vi "slowcontrol3.vi"(6 "stop":bool, 7 "VISA resource name":refnum<visa-resource-name>="COM5", 8 "Write to file":bool=TRUE, 10 "IP Address of NIST Server":string="128.210.146.230", 11 "Output Directory":path) -> (0 "data":string[](array[string]), 3 "unix time stamp":u64)   [LabVIEW 2012]
uses:
  <vilib>/Platform/TimedLoop/XDataNode/timing_clust.ctl
  <vilib>/Platform/TimedLoop/XDataNode/nitl_modes.ctl
  <vilib>/Platform/TimedLoop/XDataNode/wakeup.ctl
  <vilib>/Platform/TimedLoop/TimeConversion.llb/rt-rel-time-to-milliseconds.vi
  <vilib>/Instr/_visa.llb/VISA Configure Serial Port (Instr).vi
  <vilib>/Platform/TimedLoop/XDataNode/XDataNode.xnode
  <vilib>/Platform/TimedLoop/XDataNode/XDNodeRunTimeDep.lvlib
panel:
  out "XML String":string
  in  "Array to specify the range":dbl[][](array[numeric])=[[1657984570.0, 30.0, 105000.0, 1000.0, 1000.0, 1000.0, 700.0, 100.0, 5.0], [1342904000.0, 20.0, 95000.0, -1000.0, -1000.0, -1000.0, 650.0, 0.0, 1.0]] format="%^#_10g"
  out "data with color code":cluster{"Color Box":u32, "String":string}[](array[cluster])
  out "mean value":dbl[](array[numeric])
  in  "Period [s]":dbl=10.0
  out "number of read-out\nvariables":i32
  out "names string":string
  out "parameternames":string
  out "date/time string":string
  out "array of datanames 2":string[](array[string])
  in  "XOFF Character":u8=19 format="%.0x"
  in  "XON Character":u8=17 format="%.0x"
  out "reinitialize arduino\nread boolean":bool
  out "Magnetic Field Z Coordinate":dbl(graph)
  out "Magnetic Field Y Coordinate":dbl(graph)
  out "Magnetic Field X Coordinate":dbl(graph)
  out "Total Magnetic Field":dbl(graph)
  out "Humidity":dbl(graph)
  out "Temperature":dbl(graph)
  out "Pressure":dbl(graph)
  in  "number of iterations to\nbuild mean value":i32=5
  out "array of datanames":string[](array[string])
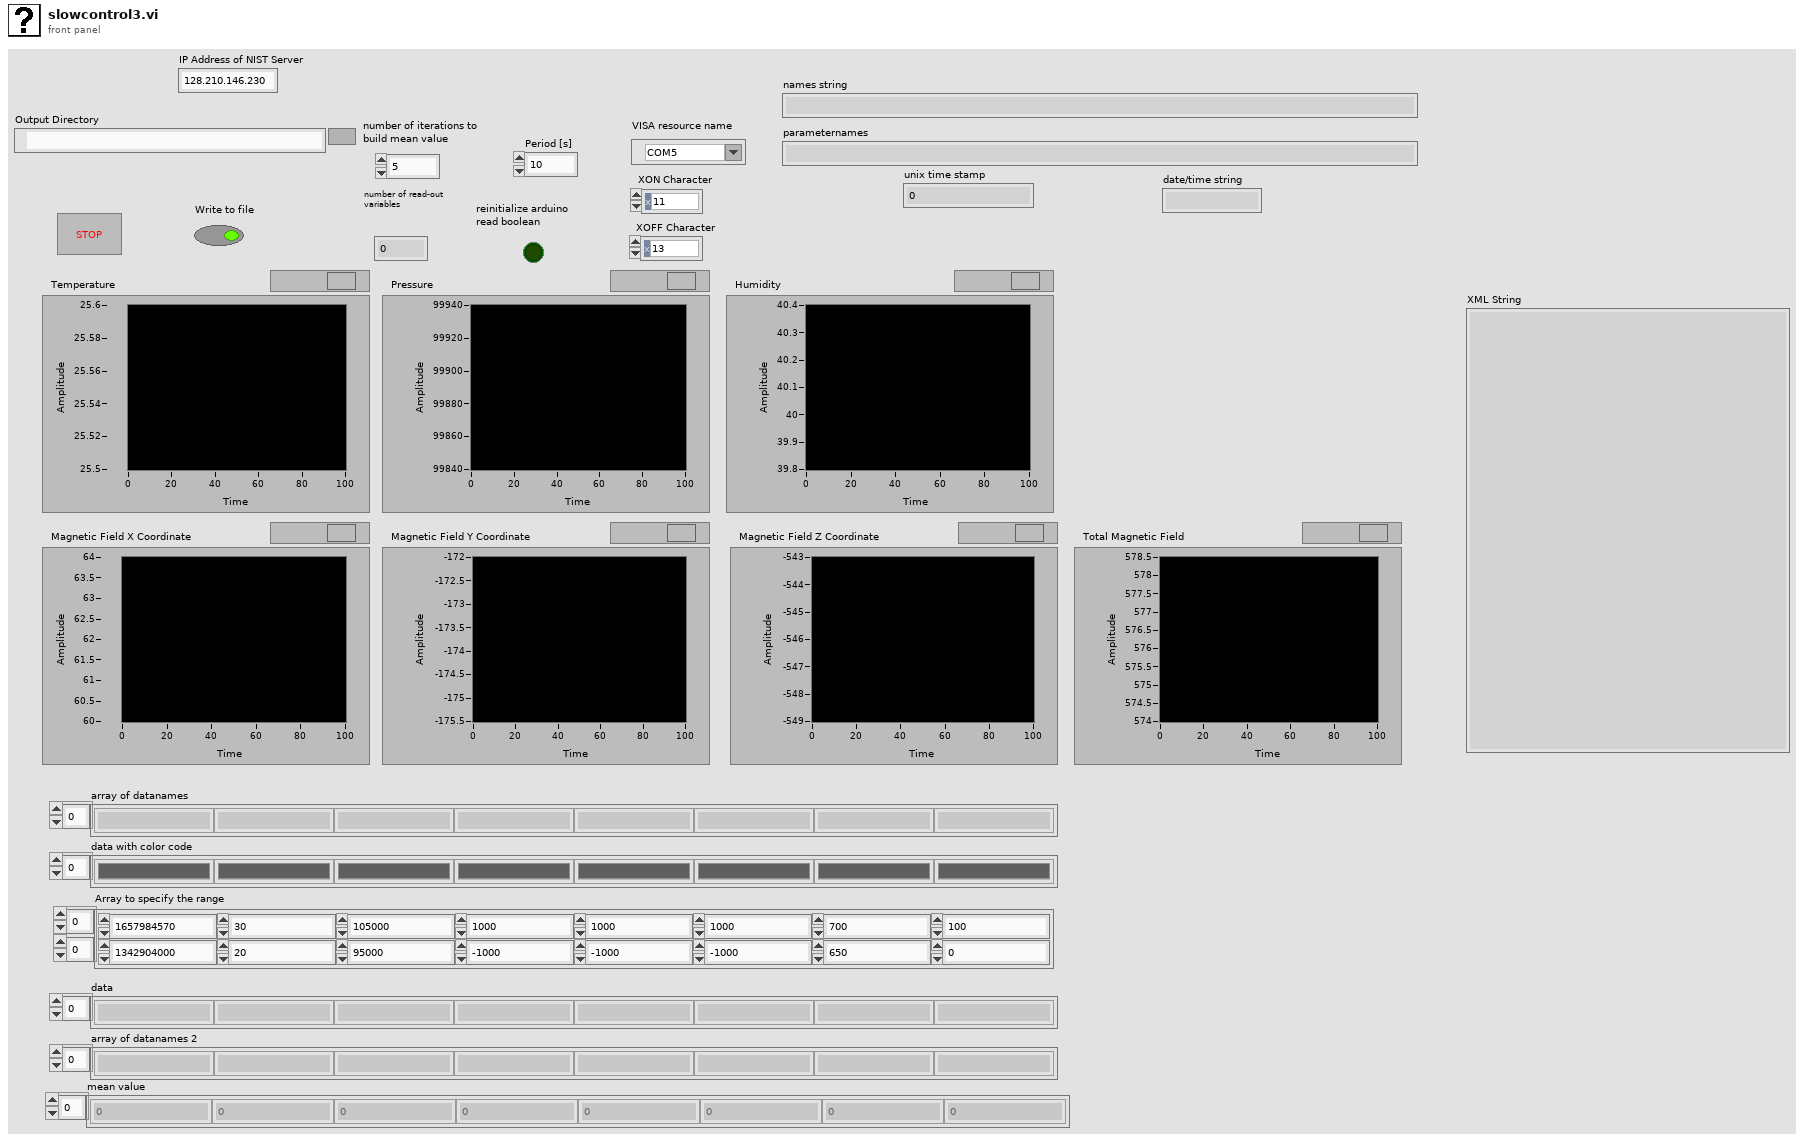
[diagram p1: front panel]
types:
  T1 = enum16{"open", "replace", "create", "open or create", "replace or create", "replace or create with confirmation"}
  T2 = typedef "XDNodeRunTimeDep.lvlib/timing_clust.ctl" = cluster{"Expected End [f-1]":u64, "Actual End [f-1]":u64, "Finished Late? [f-1]":bool, "Expected End [i-1]":u64, "Actual End [i-1]":u64, "Finished Late? [i-1]":bool, "Expected Start [i]":u64, "Actual Start [i]":u64, "Expected Start [f]":u64, "Actual Start [f]":u64, "Source Name":string, "Structure Name":string, "Period":i64, "Deadline":i64, "Offset":i64, "Start":i64, "Priority":i32, "Timeout":i32, "Mode":T3, "Wakeup Reason":T4, "Error":errorcluster, "Source Type":string, "Secondary Source Type":string, "Global End Time":u64, "Global Start Time":u64, "Frame Duration":u64, "Iteration Duration":u64, "Assigned CPU":i32, "I/O Scan Engine Mode":u32}
  T3 = typedef "XDNodeRunTimeDep.lvlib/nitl_modes.ctl" = enum32{"No Change", "Process missed periods, maintain original phase", "Discard missed periods, maintain original phase", "Process missed periods, ignore original phase", "Discard missed periods, ignore original phase"}
  T4 = typedef "XDNodeRunTimeDep.lvlib/wakeup.ctl" = enum32{"Normal", "Aborted", "Asynchronous wakeup", "Timing source error", "Timed loop error", "Timeout"}
  T5 = enum16{"big-endian, network order", "native, host order", "little-endian"}
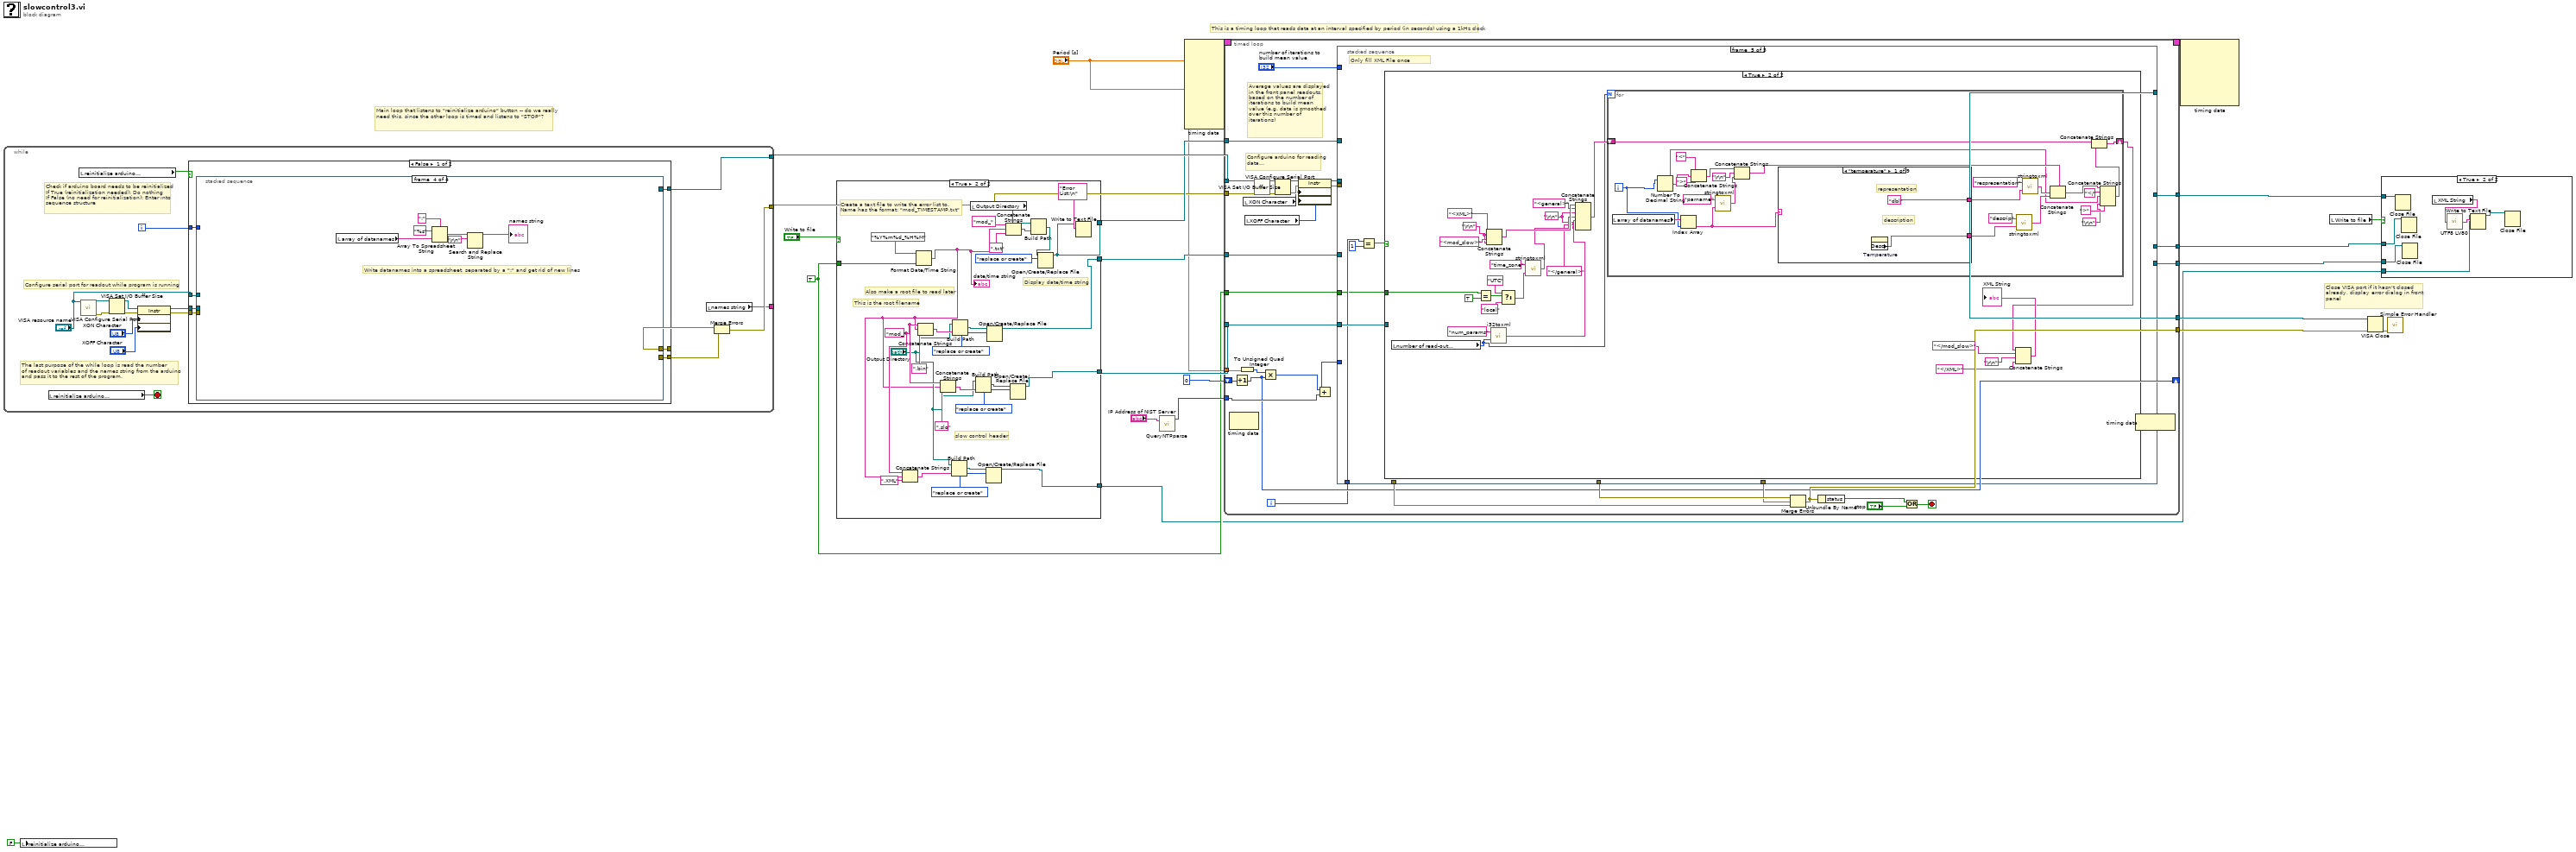
[diagram p0: block diagram]
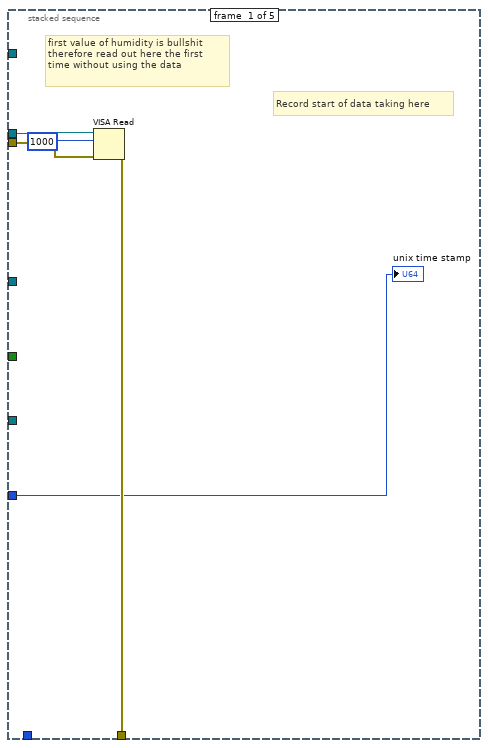
[diagram p4: hidden frame]
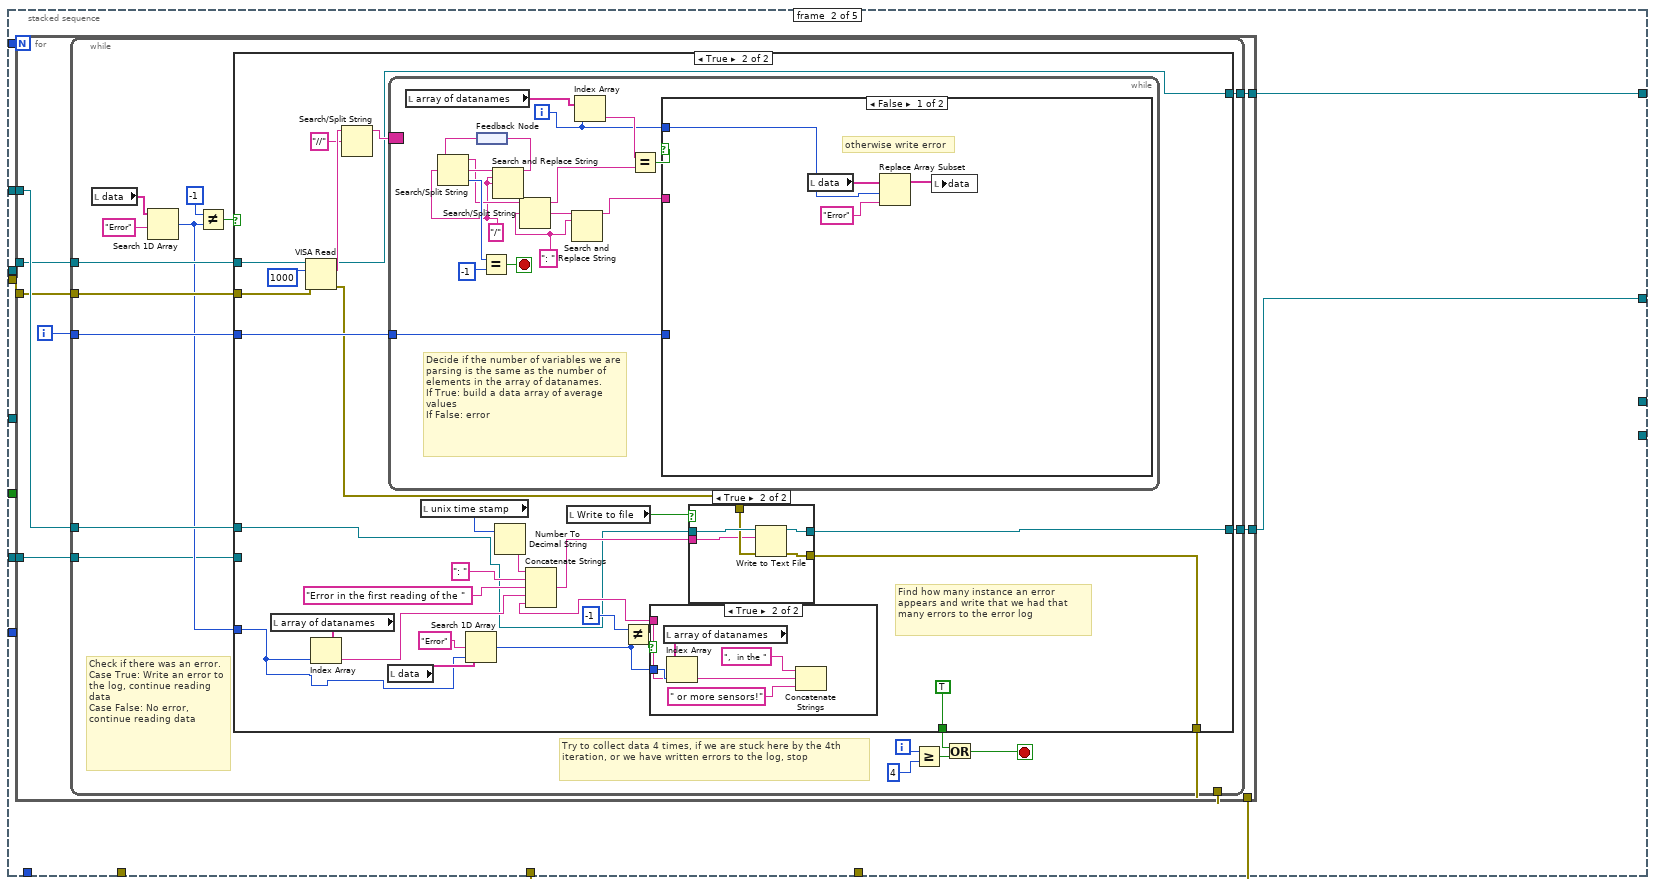
[diagram p5: hidden frame]
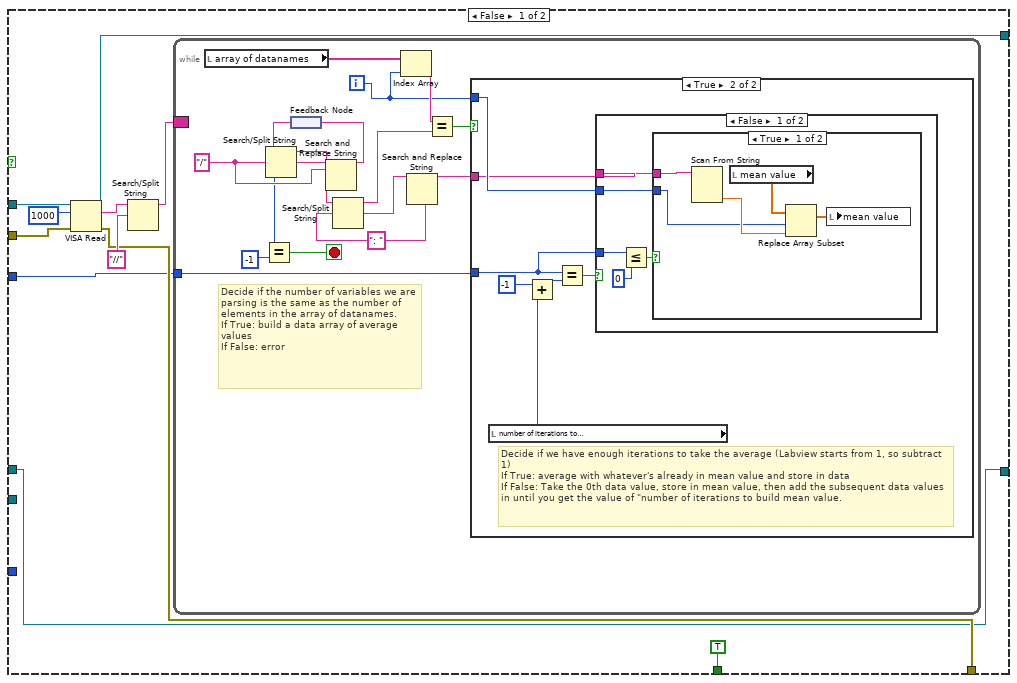
[diagram p6: hidden frame]
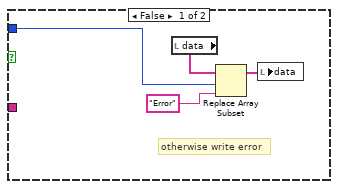
[diagram p7: hidden frame]
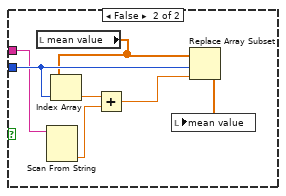
[diagram p8: hidden frame]
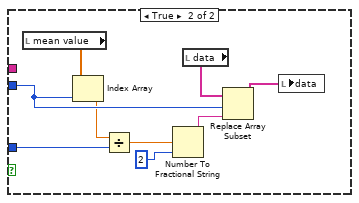
[diagram p9: hidden frame]
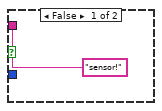
[diagram p11: hidden frame]
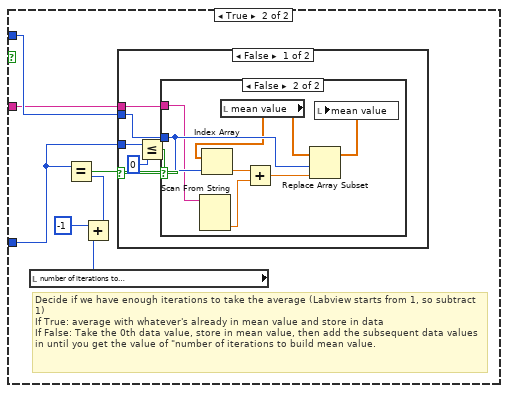
[diagram p12: hidden frame]
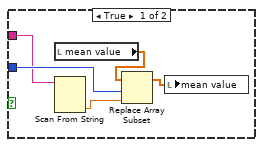
[diagram p13: hidden frame]
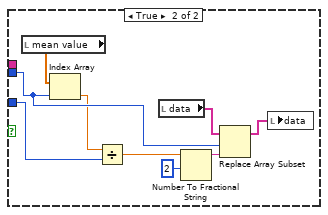
[diagram p14: hidden frame]
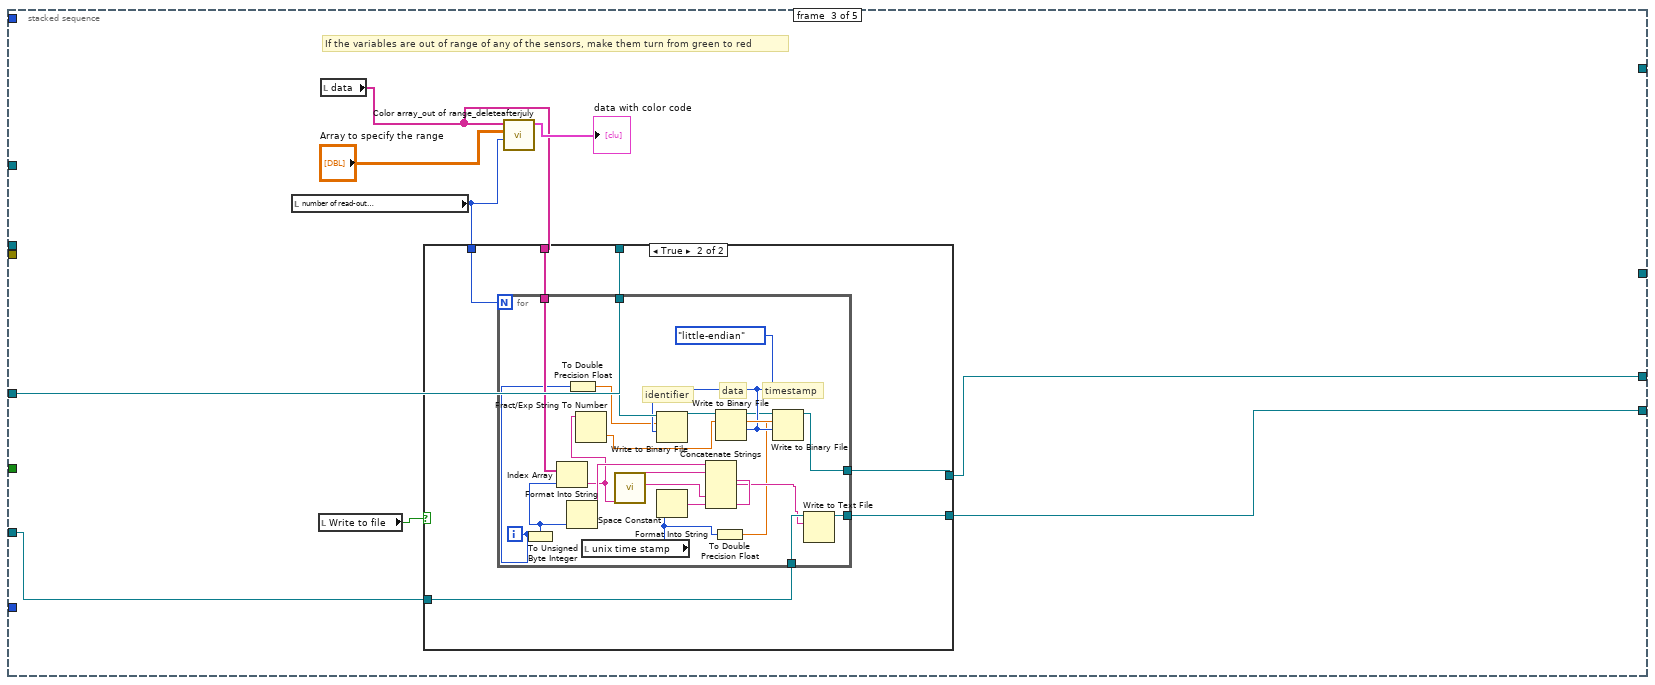
[diagram p15: hidden frame]
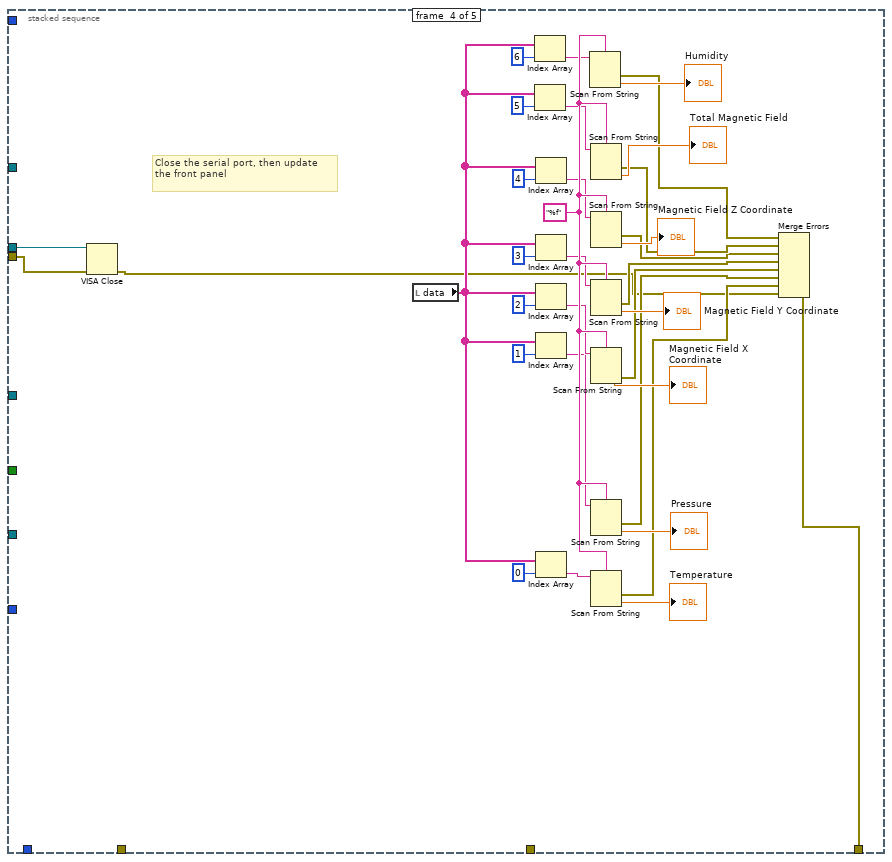
[diagram p17: hidden frame]
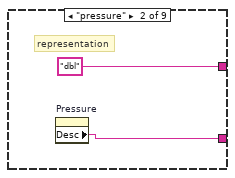
[diagram p19: hidden frame]
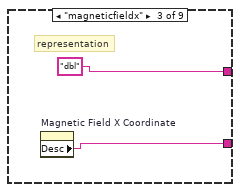
[diagram p20: hidden frame]
diagram:
  w2 = TRUE
  # "Main loop that listens to \"reinitialize arduino\" button -- do we really need this, since the other loop is timed and listens to \"STOP\"?"
  # "Close VISA port if it hasn't closed already, display error dialog in front panel"
  # "This is a timing loop that reads data at an interval specified by period (in seconds) using a 1kHz clock"
  n1 = while {
    tunnel: [w33] -> w22
    tunnel: [w32] -> w14
    tunnel: [w26] -> _
    i -> [w30]
    stop <- w28 stop-if-true
    # "The last purpose of the while loop is read the number \nof readout variables and the names string from the arduino\nand pass it to the rest of the program."
    # "Check if arduino board needs to be reinitialized\nIf True (reinitialization needed): Do nothing\nIf False (no need for reinitialization): Enter into \nsequence structure"
    # "Configure serial port for readout while program is running"
    n2 = local read "reinitialize arduino\nread boolean"() -> (w28:bool)
    n3 = local read "reinitialize arduino\nread boolean"() -> (w27:bool)
    n4 = call-poly "VISA Configure Serial Port"("VISA resource name"="VISA resource name") -> ("VISA resource name out"=w35:refnum<visa-resource-name>, "error out"=w34:errorcluster)  [unwired: 9 in, 4 out]
    n5 = VISA Set I/O Buffer Size(VISA resource name=w35, error in (no error)=w34) -> (VISA resource name out=w39:refnum<visa-resource-name>, error out=w38:errorcluster)  [unwired: 2 in]
    n6 = property class="Instr"(reference=w39, error in=w38, "Serial Settings:Flow Control XON Character"="XON Character", "Serial Settings:Flow Control XOFF Character"="XOFF Character") -> (reference out=w31:refnum<visa-resource-name>, error out=w25:errorcluster)
    n7 = case shown="False" w27 {
      tunnel: [w46 w118] -> w33
      tunnel: w31 -> [w45 w118]
      tunnel: w30 -> [w44 _]
      tunnel: "VISA resource name" -> [w43 _]
      tunnel: w25 -> [w42 _]
      tunnel: [w41 _] -> w24
      tunnel: [w40 _] -> w23
      frame False {
        n8 = stacked-sequence {
          tunnel: [_ w71 _ _] -> w46
          tunnel: w45 -> [_ w74 w91 _]
          tunnel: w44 -> [w51 _ _ _]
          tunnel: w43 -> [w48 _ _ _]
          tunnel: w42 -> [_ w72 w89 _]
          tunnel: [_ w61 _ _] -> w41
          tunnel: [_ _ w88 _] -> w40
          frame #0 {
            # "If, after 4 loop iterations, we are still here, the sensor reading must have failed??  \nSo, set the reinitialize arduino value to true and stop the program"
            # "number of runs to try to fill the array"
            n9 = Greater Or Equal?(x=w51, y=4) -> (x >= y?=w49:bool)
            n10 = case shown="True" w49 {
              tunnel: w48 -> [_ w52]
              frame False {
              }
              frame True {
                n11 = flat-sequence {
                  tunnel: w52 -> [w53]
                  frame #0 {
                    # "Report and error and close VISA"
                    n12 = VISA Close(VISA resource name=w53) -> ()  [unwired: 1 in, 1 out]
                    n13 = One Button Dialog(message="Read-out of the names of the sensors failed.\nProgram will be stopped") -> ()  [unwired: 1 in, 1 out]
                  }
                  frame #1 {
                    # "Stop the program"
                    n14 = Stop(stop? (T)=TRUE) -> ()
                  }
                }
              }
            }
            "reinitialize arduino\nread boolean" <- TRUE ("reinitialize arduino\nread boolean")
          }
          frame #1 {
            w58 = "" ("names string")
            # "The rest must be data, so there you go..."
            # "Count the number of names, \nis the number of read-out variables"
            # "Search for the \"//\" at the start of the file, \nindicates data names are here"
            # "Initialize the local variables: \nnames string\nparameternames"
            # "Read the first 1000 bytes, \noutput as a string"
            # "Initialize the array and set it to zero"
            n15 = local write "names string"(w58) -> ()
            n16 = VISA Read(VISA resource name=w74, byte count=u32 1000, error in (no error)=w72) -> (VISA resource name out=w71:refnum<visa-resource-name>, read buffer=w70:string, error out=w62:errorcluster)  [unwired: 1 out]
            n17 = Search/Split String(string=w70, search string/char (-)="//") -> (substring before match=w66:string)  [unwired: 1 in, 2 out]
            n18 = while {
              border: w66 -> [_]
              i -> [w75]
              stop <- w84 stop-if-true
              w80 = "/" ("search string/char (-)")
              # "Further separate names by \":\"'s?"
              # "When no more \"/\"s are found,\n end while loop"
              # "Names are separated by \"/\"s, so search\n for them but do not replace"
              # "Separate array names and put them into \nthe local variable \"array of datanames\""
              n19 = feedback #1() -> (w82:string)
              n20 = Search/Split String(string=w82, search string/char (-)=w80) -> (substring before match=w78:string, match + rest of string=w77:string, offset of match=w79:i32)  [unwired: 1 in]
              n21 = Search and Replace String(input string=w77, search string=w80) -> (result string=w81:string)  [unwired: 6 in, 3 out]
              n22 = feedback-in #1(w81) -> ()
              n23 = Equal?(x=w79, y=-1) -> (x = y?=w84:bool)
              n24 = Search/Split String(string=w78, search string/char (-)=": " ("format string")) -> (substring before match=w76:string)  [unwired: 1 in, 2 out]
              n25 = local read "array of datanames"() -> (w86:string[])
              n26 = Replace Array Subset(array=w86, new element=w76, index=w75) -> (w85:string[])
              n27 = local write "array of datanames"(w85) -> ()
            }
            n28 = Search and Replace String(replace all?=TRUE ("replace all? (F)"), input string=w66, search string="/", error in=w62) -> (number of replacements=w67:i32, error out=w61:errorcluster)  [unwired: 4 in, 2 out]
            n29 = Add(x=1, y=w67) -> (x+y=w57:i32)
            "number of read-out\nvariables" <- w57
            n30 = Initialize Array("", w57) -> (→"data" →"array of datanames" →"array of datanames 2":string[])
            n31 = Initialize Array(0.0 ("element"), w57) -> (→"mean value":dbl[])
            "parameternames" <- w58
          }
          frame #2 {
            # "Fill array of datanames 2 to check???\nIf they don't match, reinitialize."
            n32 = VISA Read(VISA resource name=w91, byte count=u32 1000, error in (no error)=w89) -> (read buffer=w94:string, error out=w88:errorcluster)  [unwired: 2 out]
            n33 = Search/Split String(string=w94, search string/char (-)="//") -> (substring before match=w90:string)  [unwired: 1 in, 2 out]
            n34 = while {
              border: w90 -> [_]
              i -> [w95]
              stop <- w106 stop-if-true
              w101 = "/" ("search string/char (-)")
              # "second output to manually\ncontrol the array"
              # "check if the name already exists"
              # "control the names in the array"
              n35 = local read "array of datanames 2"() -> (w108:string[])
              n36 = feedback #2() -> (w104:string)
              n37 = Search/Split String(string=w104, search string/char (-)=w101) -> (substring before match=w109:string, match + rest of string=w103:string, offset of match=w100:i32)  [unwired: 1 in]
              n38 = Search and Replace String(input string=w103, search string=w101) -> (result string=w102:string)  [unwired: 6 in, 3 out]
              n39 = feedback-in #2(w102) -> ()
              n40 = Search/Split String(string=w109, search string/char (-)=": " ("format string")) -> (substring before match=w97:string)  [unwired: 1 in, 2 out]
              n41 = Equal?(x=w100, y=-1) -> (x = y?=w106:bool)
              n42 = local read "array of datanames"() -> (w98:string[])
              n43 = Replace Array Subset(array=w108, new element=w97, index=w95) -> (w107:string[])
              n44 = local write "array of datanames 2"(w107) -> ()
              n45 = Index Array(array=w98, index=w95) -> (element=w99:string)
              n46 = Equal?(x=w99, y=w97) -> (x = y?=w96:bool)
              n47 = case shown="False" w96 {
                frame False {
                  n48 = local write "reinitialize arduino\nread boolean"(FALSE ("reinitialize arduino read boolean")) -> ()
                }
                frame True {
                }
              }
            }
          }
          frame #3 {
            # "Write datanames into a spreadsheet, separated by a \":\" and get rid of new lines"
            n49 = local read "array of datanames"() -> (w117:string[])
            n50 = Array To Spreadsheet String(delimiter (Tab)=":", array=w117, 3:"%s" ("format string")) -> (spreadsheet string=w113:string)
            n51 = Search and Replace String(input string=w113, search string="\r\n") -> (result string=→"names string":string)  [unwired: 6 in, 3 out]
          }
        }
      }
      frame True {
      }
    }
    n52 = local read "names string"() -> (w26:string)
    n53 = Merge Errors(w24, w23) -> (w32:errorcluster)
  }
  n54 = local write "reinitialize arduino\nread boolean"(FALSE ("reinitialize arduino\nread boolean")) -> ()
  n55 = case shown="True" "Write to file" {
    tunnel: [_ w141] -> w18
    tunnel: [_ w130] -> w13
    tunnel: [_ w129] -> w4
    tunnel: [_ w122] -> w1
    tunnel: w2 -> [_ w119]
    frame False {
    }
    frame True {
      w126 = "mod_"
      # "slow control header"
      # "This is the root filename"
      # "Display date/time string"
      # "Also make a root file to read later"
      # "Create a text file to write the error list to.  \nName has the format: \"mod_TIMESTAMP.txt\""
      n56 = Format Date/Time String(time format string (%c)="%Y%m%d_%H%M", UTC format=w119) -> (date/time string=w120:string)  [unwired: 1 in]
      "date/time string" <- w120
      n57 = Concatenate Strings(w126, w120, ".XML" ("string")) -> (w124:string)
      n58 = Concatenate Strings(w126, w120, ".bin") -> (w139:string)
      n59 = Concatenate Strings(w126, w120, ".slo") -> (w131:string)
      n60 = Build Path(base path="Output Directory", name or relative path=w124) -> (appended path=w127:path)
      n61 = Build Path(base path="Output Directory", name or relative path=w139) -> (appended path=w138:path)
      n62 = local read "Output Directory"() -> (w137:path)
      n63 = Build Path(base path="Output Directory", name or relative path=w131) -> (appended path=w132:path)
      n64 = Open/Create/Replace File(file path (use dialog)=w127, operation (0:open)=T1."replace or create") -> (refnum out=w122:refnum<file>)  [unwired: 4 in, 2 out]
      n65 = Open/Create/Replace File(file path (use dialog)=w138, operation (0:open)=T1."replace or create") -> (refnum out=w130:refnum<file>)  [unwired: 4 in, 2 out]
      n66 = Concatenate Strings("mod_", w120, ".txt") -> (w136:string)
      n67 = Open/Create/Replace File(file path (use dialog)=w132, operation (0:open)=T1."replace or create") -> (refnum out=w129:refnum<file>)  [unwired: 4 in, 2 out]
      n68 = Build Path(base path=w137, name or relative path=w136) -> (appended path=w135:path)
      n69 = Open/Create/Replace File(file path (use dialog)=w135, operation (0:open)=T1."replace or create") -> (refnum out=w141:refnum<file>)  [unwired: 4 in, 2 out]
      n70 = Write to Text File(file (use dialog)=w141, text="Error List:\n") -> ()  [unwired: 2 in, 3 out]
    }
  }
  n71 = call "QueryNTPparse.vi"("Hostname"="IP Address of NIST Server") -> ("NTP Time"=w5:u64)  [unwired: 1 in, 2 out]
  n72 = node-c288("Period [s]") -> (w21:T2)  [unwired: 9 in]
  n73 = timed-loop {
    tunnel: w22 -> [w173]
    tunnel: w14 -> [w171]
    tunnel: [w174] -> w15
    timing: w21 -> [_]
    timing-out: [_] -> w20
    tunnel: w18 -> [w175]
    tunnel: [w163] -> w16
    tunnel: w13 -> [w160]
    tunnel: [w149] -> w12
    tunnel: [w159] -> w11
    tunnel: w5 -> [w157]
    shift-right: [w152] -> _
    shift-left: u64 0 -> [w158]
    tunnel: "Period [s]" -> [w155]
    tunnel: w4 -> [w151]
    tunnel: [w150] -> w3
    tunnel: w2 -> [w147]
    i -> [w148]
    stop <- w178 stop-if-true
    # "Configure arduino for reading data..."
    # "Average values are displayed in the front panel readouts, based on the number of iterations to build mean value (e.g. data is smoothed over this number of iterations)"
    n74 = node-c288() -> ()  [unwired: 1 in, 1 out]
    n75 = Increment(x=w158) -> (x+1=w152:u64)
    n76 = To Unsigned Quad Integer(1:w155) -> (0:w154:u64)
    n77 = local read "XON Character"() -> (w164:u8)
    n78 = local read "XOFF Character"() -> (w165:u8)
    n79 = call-poly "VISA Configure Serial Port"("VISA resource name"=w173, "error in (no error)"=w171) -> ("VISA resource name out"=w172:refnum<visa-resource-name>, "error out"=w170:errorcluster)  [unwired: 8 in, 4 out]
    n80 = Multiply(x=w154, y=w152) -> (x*y=w153:u64)
    n81 = VISA Set I/O Buffer Size(VISA resource name=w172, error in (no error)=w170) -> (VISA resource name out=w166:refnum<visa-resource-name>, error out=w169:errorcluster)  [unwired: 2 in]
    n82 = property class="Instr"(reference=w166, error in=w169, "Serial Settings:Flow Control XON Character"=w164, "Serial Settings:Flow Control XOFF Character"=w165) -> (reference out=w167:refnum<visa-resource-name>, error out=w168:errorcluster)
    n83 = Add(x=w153, y=w157) -> (x+y=w156:u64)
    n84 = stacked-sequence {
      tunnel: [_ _ _ w420 _] -> w176
      tunnel: [_ w192 _ _ _] -> w177
      tunnel: w175 -> [_ w193 _ _ _]
      tunnel: w168 -> [w186 w195 _ w418 _]
      tunnel: w167 -> [w187 w194 _ w419 _]
      tunnel: [_ w191 _ _ _] -> w163
      tunnel: "number of iterations to\nbuild mean value" -> [_ w190 _ _ _]
      tunnel: [w184 _ _ _ _] -> w161
      tunnel: w160 -> [_ _ w388 _ _]
      tunnel: [_ _ w389 _ _] -> w159
      tunnel: w156 -> [w183 _ _ _ _]
      tunnel: w151 -> [_ w189 w384 _ w455]
      tunnel: [_ _ w383 _ _] -> w150
      tunnel: [_ w188 _ _ _] -> w149
      tunnel: w148 -> [_ _ _ _ w453]
      tunnel: w147 -> [_ _ _ _ w451]
      frame #0 {
        # "first value of humidity is bullshit therefore read out here the first time without using the data"
        # "Record start of data taking here"
        n85 = VISA Read(VISA resource name=w187, byte count=u32 1000, error in (no error)=w186) -> (error out=w184:errorcluster)  [unwired: 3 out]
        "unix time stamp" <- w183
      }
      frame #1 {
        n86 = for {
          N: w190 -> [_]
          tunnel: w195 -> [w200]
          tunnel: w194 -> [w201]
          tunnel: w193 -> [w203]
          tunnel: [w202] -> w192
          tunnel: [w199] -> w191
          tunnel: [w197] -> w188
          tunnel: w189 -> [w196]
          i -> [w198]
          n87 = while {
            tunnel: w203 -> [w215]
            tunnel: [w214] -> w202
            tunnel: w201 -> [w213]
            tunnel: w200 -> [w211]
            tunnel: [w212] -> w199
            tunnel: w198 -> [w210]
            tunnel: [w207] -> w197
            tunnel: w196 -> [w204]
            i -> [w220]
            stop <- w216 stop-if-true
            # "Try to collect data 4 times, if we are stuck here by the 4th iteration, or we have written errors to the log, stop"
            # "Check if there was an error.  \nCase True: Write an error to the log, continue reading data\nCase False: No error, continue reading data"
            n88 = local read "data"() -> (w206:string[])
            n89 = Search 1D Array(1D array=w206, element="Error") -> (index of element=w208:i32)  [unwired: 1 in]
            n90 = Not Equal?(x=-1 ("y"), y=w208) -> (x != y?=w205:bool)
            n91 = case shown="True" w205 {
              tunnel: w208 -> [_ w289]
              tunnel: [TRUE TRUE] -> w217
              tunnel: w215 -> [w222 w297]
              tunnel: [w224 w296] -> w214
              tunnel: w213 -> [w227 w295]
              tunnel: [w226 w294] -> w212
              tunnel: w211 -> [w225 w293]
              tunnel: w210 -> [w223 w292]
              tunnel: [w222 w290] -> w207
              tunnel: w204 -> [_ _]
              frame False {
                n92 = VISA Read(VISA resource name=w227, byte count=u32 1000, error in (no error)=w225) -> (VISA resource name out=w226:refnum<visa-resource-name>, read buffer=w228:string, error out=w224:errorcluster)  [unwired: 1 out]
                n93 = Search/Split String(string=w228, search string/char (-)="//") -> (substring before match=w231:string)  [unwired: 1 in, 2 out]
                n94 = while {
                  border: w231 -> [_]
                  tunnel: w223 -> [w234]
                  i -> [w233]
                  stop <- w249 stop-if-true
                  w237 = ": " ("format string")
                  w244 = "/" ("search string/char (-)")
                  # "Decide if the number of variables we are parsing is the same as the number of elements in the array of datanames.  \nIf True: build a data array of average values\nIf False: error"
                  n95 = local read "array of datanames"() -> (w240:string[])
                  n96 = feedback #3() -> (w247:string)
                  n97 = Search/Split String(string=w247, search string/char (-)=w244) -> (substring before match=w238:string, match + rest of string=w246:string, offset of match=w243:i32)  [unwired: 1 in]
                  n98 = Equal?(x=w243, y=-1) -> (x = y?=w249:bool)
                  n99 = Search and Replace String(input string=w246, search string=w244) -> (result string=w245:string)  [unwired: 6 in, 3 out]
                  n100 = feedback-in #3(w245) -> ()
                  n101 = Search/Split String(string=w238, search string/char (-)=w237) -> (substring before match=w242:string, match + rest of string=w239:string)  [unwired: 1 in, 1 out]
                  n102 = Index Array(array=w240, index=w233) -> (element=w241:string)
                  n103 = Search and Replace String(input string=w239, search string=w237) -> (result string=w235:string)  [unwired: 6 in, 3 out]
                  n104 = Equal?(x=w241, y=w242) -> (x = y?=w236:bool)
                  n105 = case shown="True" w236 {
                    tunnel: w235 -> [_ w259]
                    tunnel: w233 -> [w253 w260]
                    tunnel: w234 -> [_ w257]
                    frame False {
                      # "otherwise write error"
                      n106 = local read "data"() -> (w252:string[])
                      n107 = Replace Array Subset(array=w252, new element="Error" ("new element/subarray"), index=w253) -> (w251:string[])
                      n108 = local write "data"(w251) -> ()
                    }
                    frame True {
                      # "Decide if we have enough iterations to take the average (Labview starts from 1, so subtract 1)\nIf True: average with whatever's already in mean value and store in data\nIf False: Take the 0th data value, store in mean value, then add the subsequent data values in until you get the value of \"number of iterations to build mean value."
                      n109 = local read "number of iterations to\nbuild mean value"() -> (w256:i32)
                      n110 = Add(x=-1, y=w256) -> (x+y=w255:i32)
                      n111 = Equal?(x=w257, y=w255) -> (x = y?=w258:bool)
                      n112 = case shown="False" w258 {
                        tunnel: w257 -> [w265 w282]
                        tunnel: w260 -> [w262 w285]
                        tunnel: w259 -> [w261 _]
                        frame False {
                          n113 = Less Or Equal?(x=w265, y=0) -> (x <= y?=w264:bool)
                          n114 = case shown="True" w264 {
                            tunnel: w262 -> [w266 w276]
                            tunnel: w261 -> [w270 w275]
                            frame True {
                              n115 = Scan From String(input string=w270) -> (output 1=w269:dbl)  [unwired: 4 in, 3 out]
                              n116 = local read "mean value"() -> (w268:dbl[])
                              n117 = Replace Array Subset(array=w268, new element=w269, index=w266) -> (w267:dbl[])
                              n118 = local write "mean value"(w267) -> ()
                            }
                            frame False {
                              n119 = local read "mean value"() -> (w271:dbl[])
                              n120 = Scan From String(input string=w275) -> (output 1=w274:dbl)  [unwired: 4 in, 3 out]
                              n121 = Index Array(array=w271, index=w276) -> (element=w272:dbl)
                              n122 = Add(x=w272, y=w274) -> (x+y=w273:dbl)
                              n123 = Replace Array Subset(array=w271, new element=w273, index=w276) -> (w277:dbl[])
                              n124 = local write "mean value"(w277) -> ()
                            }
                          }
                        }
                        frame True {
                          n125 = local read "mean value"() -> (w279:dbl[])
                          n126 = Index Array(array=w279, index=w285) -> (element=w278:dbl)
                          n127 = Divide(x=w278, y=w282) -> (x/y=w283:dbl)
                          n128 = Number To Fractional String(number=w283, precision (6)=i16 2) -> (F-format string=w286:string)  [unwired: 2 in]
                          n129 = local read "data"() -> (w284:string[])
                          n130 = Replace Array Subset(array=w284, new element=w286, index=w285) -> (w281:string[])
                          n131 = local write "data"(w281) -> ()
                        }
                      }
                    }
                  }
                }
              }
              frame True {
                # "Find how many instance an error appears and write that we had that many errors to the error log"
                n132 = local read "array of datanames"() -> (w307:string[])
                n133 = VISA Read(VISA resource name=w295, byte count=u32 1000, error in (no error)=w293) -> (VISA resource name out=w294:refnum<visa-resource-name>, read buffer=w314:string, error out=w291:errorcluster)  [unwired: 1 out]
                n134 = Index Array(array=w307, index=w289) -> (element=w306:string)
                n135 = Search/Split String(string=w314, search string/char (-)="//") -> (substring before match=w311:string)  [unwired: 1 in, 2 out]
                n136 = local read "data"() -> (w305:string[])
                n137 = while {
                  border: w311 -> [_]
                  tunnel: w292 -> [w331]
                  i -> [w329]
                  stop <- w345 stop-if-true
                  w332 = ": " ("format string")
                  w330 = "/" ("search string/char (-)")
                  # "Decide if the number of variables we are parsing is the same as the number of elements in the array of datanames.  \nIf True: build a data array of average values\nIf False: error"
                  n138 = local read "array of datanames"() -> (w335:string[])
                  n139 = feedback #4() -> (w343:string)
                  n140 = Search/Split String(string=w343, search string/char (-)=w330) -> (substring before match=w333:string, match + rest of string=w342:string, offset of match=w340:i32)  [unwired: 1 in]
                  n141 = Equal?(x=w340, y=-1) -> (x = y?=w345:bool)
                  n142 = Search and Replace String(input string=w342, search string=w330, replace string=w330) -> (result string=w341:string)  [unwired: 5 in, 3 out]
                  n143 = feedback-in #4(w341) -> ()
                  n144 = Search/Split String(string=w333, search string/char (-)=w332) -> (substring before match=w338:string, match + rest of string=w334:string)  [unwired: 1 in, 1 out]
                  n145 = Search and Replace String(input string=w334, search string=w332) -> (result string=w339:string)  [unwired: 6 in, 3 out]
                  n146 = Index Array(array=w335, index=w329) -> (element=w337:string)
                  n147 = Equal?(x=w337, y=w338) -> (x = y?=w336:bool)
                  n148 = case shown="False" w336 {
                    tunnel: w339 -> [_ w355]
                    tunnel: w329 -> [w349 w356]
                    tunnel: w331 -> [_ w353]
                    frame False {
                      # "otherwise write error"
                      n149 = local read "data"() -> (w348:string[])
                      n150 = Replace Array Subset(array=w348, new element="Error" ("new element/subarray"), index=w349) -> (w347:string[])
                      n151 = local write "data"(w347) -> ()
                    }
                    frame True {
                      # "Decide if we have enough iterations to take the average (Labview starts from 1, so subtract 1)\nIf True: average with whatever's already in mean value and store in data\nIf False: Take the 0th data value, store in mean value, then add the subsequent data values in until you get the value of \"number of iterations to build mean value."
                      n152 = local read "number of iterations to\nbuild mean value"() -> (w352:i32)
                      n153 = Add(x=-1, y=w352) -> (x+y=w351:i32)
                      n154 = Equal?(x=w353, y=w351) -> (x = y?=w354:bool)
                      n155 = case shown="False" w354 {
                        tunnel: w353 -> [w361 w380]
                        tunnel: w356 -> [w358 w382]
                        tunnel: w355 -> [w357 _]
                        frame False {
                          n156 = Less Or Equal?(x=w361, y=0) -> (x <= y?=w360:bool)
                          n157 = case shown="False" w360 {
                            tunnel: w358 -> [w363 w372]
                            tunnel: w357 -> [w362 w371]
                            frame True {
                              n158 = local read "mean value"() -> (w365:dbl[])
                              n159 = Scan From String(input string=w362) -> (output 1=w366:dbl)  [unwired: 4 in, 3 out]
                              n160 = Replace Array Subset(array=w365, new element=w366, index=w363) -> (w364:dbl[])
                              n161 = local write "mean value"(w364) -> ()
                            }
                            frame False {
                              n162 = Scan From String(input string=w371) -> (output 1=w370:dbl)  [unwired: 4 in, 3 out]
                              n163 = local read "mean value"() -> (w367:dbl[])
                              n164 = Index Array(array=w367, index=w372) -> (element=w369:dbl)
                              n165 = Add(x=w369, y=w370) -> (x+y=w368:dbl)
                              n166 = Replace Array Subset(array=w367, new element=w368, index=w372) -> (w373:dbl[])
                              n167 = local write "mean value"(w373) -> ()
                            }
                          }
                        }
                        frame True {
                          n168 = local read "mean value"() -> (w374:dbl[])
                          n169 = Index Array(array=w374, index=w382) -> (element=w376:dbl)
                          n170 = Divide(x=w376, y=w380) -> (x/y=w375:dbl)
                          n171 = local read "data"() -> (w381:string[])
                          n172 = Number To Fractional String(number=w375, precision (6)=i16 2) -> (F-format string=w378:string)  [unwired: 2 in]
                          n173 = Replace Array Subset(array=w381, new element=w378, index=w382) -> (w379:string[])
                          n174 = local write "data"(w379) -> ()
                        }
                      }
                    }
                  }
                }
                n175 = local read "unix time stamp"() -> (w287:u64)
                n176 = Search 1D Array(1D array=w305, element="Error", start index (0)=w289) -> (index of element=w301:i32)
                n177 = Number To Decimal String(number=w287) -> (decimal integer string=w310:string)  [unwired: 1 in]
                n178 = local read "Write to file"() -> (w288:bool)
                n179 = Not Equal?(x=-1 ("y"), y=w301) -> (x != y?=w303:bool)
                n180 = case shown="True" w303 {
                  tunnel: w301 -> [_ w327]
                  tunnel: ["sensor!" w323] -> w300
                  frame False {
                  }
                  frame True {
                    n181 = local read "array of datanames"() -> (w328:string[])
                    n182 = Index Array(array=w328, index=w327) -> (element=w325:string)
                    n183 = Concatenate Strings(",  in the " ("string"), w325, " or more sensors!" ("string")) -> (w323:string)
                  }
                }
                n184 = Concatenate Strings(w310, ": ", "Error in the first reading of the ", w306, w300) -> (w299:string)
                n185 = case shown="True" w288 {
                  tunnel: w299 -> [_ w317]
                  tunnel: w297 -> [w316 w321]
                  tunnel: [w315 w320] -> w296
                  tunnel: w291 -> [w315 w319]
                  tunnel: [w316 w318] -> w290
                  frame False {
                  }
                  frame True {
                    n186 = Write to Text File(file (use dialog)=w321, text=w317, error in=w319) -> (refnum out=w318:refnum<file>, error out=w320:errorcluster)  [unwired: 1 in, 1 out]
                  }
                }
              }
            }
            n187 = Greater Or Equal?(x=w220, y=4) -> (x >= y?=w218:bool)
            n188 = Or(x=w217, y=w218) -> (x .or. y?=w216:bool)
          }
        }
      }
      frame #2 {
        # "If the variables are out of range of any of the sensors, make them turn from green to red"
        n189 = local read "number of read-out\nvariables"() -> (w386:i32)
        n190 = local read "Write to file"() -> (w385:bool)
        n191 = local read "data"() -> (w387:string[])
        n192 = case shown="True" w385 {
          tunnel: [_ w397] -> w389
          tunnel: w388 -> [_ w396]
          tunnel: w387 -> [_ w395]
          tunnel: w386 -> [_ w394]
          tunnel: [_ w393] -> w383
          tunnel: w384 -> [_ w392]
          frame False {
          }
          frame True {
            n193 = for {
              N: w394 -> [_]
              tunnel: [w400] -> w397
              tunnel: w396 -> [w409]
              tunnel: w395 -> [w416]
              tunnel: [w411] -> w393
              tunnel: w392 -> [w410]
              i -> [w402]
              w405 = T5."little-endian" ("byte order (0:big-endian, network order)")
              # "timestamp"
              # "data"
              # "identifier"
              n194 = To Unsigned Byte Integer(number=w402) -> (unsigned 8bit integer=w412:u8)
              n195 = Index Array(array=w416, index=w412) -> (element=w408:string)
              n196 = Format Into String(w412) -> (resulting string=w415:string)  [unwired: 3 in, 1 out]
              n197 = To Double Precision Float(number=w402) -> (double precision float=w401:dbl)
              n198 = Fract/Exp String To Number(string=w408) -> (number=w407:dbl)  [unwired: 3 in, 1 out]
              n199 = local read "unix time stamp"() -> (w404:u64)
              n200 = call <vilib>:"Space Constant.vi"() -> ("String"=w413:string)
              n201 = Write to Binary File(file (use dialog)=w409, data=w401, 9:w405) -> (refnum out=w398:refnum<file>)  [unwired: 3 in, 2 out]
              n202 = Format Into String(w404) -> (resulting string=w414:string)  [unwired: 3 in, 1 out]
              n203 = Concatenate Strings(w415, w413, w414, w413, w408, w413) -> (w406:string)
              n204 = To Double Precision Float(number=w404) -> (double precision float=w403:dbl)
              n205 = Write to Binary File(file (use dialog)=w398, data=w403, 9:w405) -> (refnum out=w399:refnum<file>)  [unwired: 3 in, 2 out]
              n206 = Write to Binary File(file (use dialog)=w399, data=w407, 9:w405) -> (refnum out=w400:refnum<file>)  [unwired: 3 in, 2 out]
              n207 = Write to Text File(file (use dialog)=w410, text=w406) -> (refnum out=w411:refnum<file>)  [unwired: 2 in, 2 out]
            }
          }
        }
        n208 = call "Color array_out of range_deleteafterjuly.vi"("Number of sensors"=w386, "Array to specify\nthe range"="Array to specify the range", "Input Array"=w387) -> ("output array with color code"=→"data with color code":cluster{"Color Box":u32, "String":string}[])  [unwired: 7 in, 1 out]
      }
      frame #3 {
        w434 = "%f" ("format string")
        # "Close the serial port, then update the front panel"
        n209 = VISA Close(VISA resource name=w419, error in (no error)=w418) -> (error out=w417:errorcluster)
        n210 = local read "data"() -> (w443:string[])
        n211 = Index Array(array=w443, index=6) -> (element=w428:string)
        n212 = Index Array(array=w443, index=5) -> (element=w429:string)
        n213 = Index Array(array=w443, index=4) -> (element=w433:string)
        n214 = Index Array(array=w443, index=3) -> (element=w432:string)
        n215 = Index Array(array=w443, index=2) -> (element=w431:string)
        n216 = Index Array(array=w443, index=1) -> (element=w430:string)
        n217 = Index Array(array=w443, index=0) -> (element=w442:string)
        n218 = Scan From String(format string=w434, input string=w428) -> (error out=w427:errorcluster, output 1=→"Humidity":dbl)  [unwired: 3 in, 2 out]
        n219 = Scan From String(format string=w434, input string=w429) -> (error out=w426:errorcluster, output 1=→"Total Magnetic Field":dbl)  [unwired: 3 in, 2 out]
        n220 = Scan From String(format string=w434, input string=w433) -> (error out=w425:errorcluster, output 1=→"Magnetic Field Z Coordinate":dbl)  [unwired: 3 in, 2 out]
        n221 = Scan From String(format string=w434, input string=w432) -> (error out=w424:errorcluster, output 1=→"Magnetic Field Y Coordinate":dbl)  [unwired: 3 in, 2 out]
        n222 = Scan From String(format string=w434, input string=w431) -> (error out=w423:errorcluster, output 1=→"Magnetic Field X Coordinate":dbl)  [unwired: 3 in, 2 out]
        n223 = Scan From String(format string=w434, input string=w430) -> (error out=w422:errorcluster, output 1=→"Pressure":dbl)  [unwired: 3 in, 2 out]
        n224 = Scan From String(format string=w434, input string=w442) -> (error out=w421:errorcluster, output 1=→"Temperature":dbl)  [unwired: 3 in, 2 out]
        n225 = Merge Errors(w427, w426, w425, w424, w423, w422, w421, w417) -> (w420:errorcluster)
      }
      frame #4 {
        # "Only fill XML File once"
        n226 = Equal?(x=w453, y=1) -> (x = y?=w452:bool)
        n227 = case shown="True" w452 {
          tunnel: w455 -> [_ _]
          tunnel: w451 -> [_ w456]
          frame False {
          }
          frame True {
            w459 = "\r\n"
            w465 = "\r\n"
            n228 = local read "number of read-out\nvariables"() -> (w467:i32)
            n229 = Equal?(x=w456, y=TRUE) -> (x = y?=w475:bool)
            n230 = Concatenate Strings("<XML>", w465, "<mod_slow>", w465) -> (w464:string)
            n231 = call "i32toxml.vi"("variable"=w467, "variable name"="num_params") -> ("xml string"=w461:string)
            n232 = Select(t="UTC" ("XML Tag"), s=w475, f="local") -> (s? t:f=w478:string)
            n233 = call "stringtoxml.vi"("String to write"=w478, "XML Tag"="time_zone") -> ("xml string"=w462:string)
            n234 = Concatenate Strings(w464, "<general>", w459, w462, w461, "</general>" ("string"), w459) -> (w471:string)
            n235 = for {
              N: w467 -> [_]
              shift-right: [w485] -> w468
              shift-left: w471 -> [w503]
              i -> [w484]
              n236 = local read "array of datanames"() -> (w499:string[])
              n237 = Number To Decimal String(number=w484) -> (decimal integer string=w488:string)  [unwired: 1 in]
              n238 = Index Array(array=w499, index=w484) -> (element=w497:string)
              n239 = Concatenate Strings("<" ("string"), w488, ">" ("string")) -> (w500:string)
              n240 = call "stringtoxml.vi"("String to write"=w497, "XML Tag"="parname") -> ("xml string"=w482:string)
              n241 = Concatenate Strings(w500, "\r\n", w482) -> (w492:string)
              n242 = case shown="\"temperature\"" w497 {
                tunnel: ["dbl" ("XML Tag") "dbl" ("XML Tag") "dbl" ("XML Tag") "dbl" ("XML Tag") "dbl" ("XML Tag") "dbl" ("XML Tag") "dbl" ("XML Tag") "dbl" ("XML Tag") "none" ("XML Tag")] -> w494
                tunnel: [w504 w506 w508 w510 w512 w514 w516 "Number of seconds elapsed since arduino began running" ("XML Tag") "This parameter was not specified by the labview program" ("XML Tag")] -> w493
                frame "temperature" {
                  # "description"
                  # "representation"
                  n243 = property on="Temperature" class="WFChart (strict)"() -> ("Desc"=w504:string)  [unwired: 2 in, 2 out]
                }
                frame "pressure" {
                  # "representation"
                  n244 = property on="Pressure" class="WFChart (strict)"() -> ("Desc"=w506:string)  [unwired: 2 in, 2 out]
                }
                frame "magneticfieldx" {
                  # "representation"
                  n245 = property on="Magnetic Field X Coordinate" class="WFChart (strict)"() -> ("Desc"=w508:string)  [unwired: 2 in, 2 out]
                }
                frame "magneticfieldy" {
                  # "representation"
                  n246 = property on="Magnetic Field Y Coordinate" class="WFChart (strict)"() -> ("Desc"=w510:string)  [unwired: 2 in, 2 out]
                }
                frame "magneticfieldz" {
                  # "representation"
                  n247 = property on="Magnetic Field Z Coordinate" class="WFChart (strict)"() -> ("Desc"=w512:string)  [unwired: 2 in, 2 out]
                }
                frame "magneticfieldtotal" {
                  # "representation"
                  n248 = property on="Total Magnetic Field" class="WFChart (strict)"() -> ("Desc"=w514:string)  [unwired: 2 in, 2 out]
                }
                frame "humidity" {
                  # "representation"
                  n249 = property on="Humidity" class="WFChart (strict)"() -> ("Desc"=w516:string)  [unwired: 2 in, 2 out]
                }
                frame "seconds" {
                  # "representation"
                }
                frame "ERROR", Default {
                  # "representation"
                }
              }
              n250 = call "stringtoxml.vi"("String to write"=w493, "XML Tag"="descrip") -> ("xml string"=w490:string)
              n251 = call "stringtoxml.vi"("String to write"=w494, "XML Tag"="respresentation") -> ("xml string"=w491:string)
              n252 = Concatenate Strings(w492, w491, w490) -> (w480:string)
              n253 = Concatenate Strings(w480, "</" ("string"), w488, ">" ("string"), "\r\n") -> (w486:string)
              n254 = Concatenate Strings(w503, w486) -> (w485:string)
            }
            n255 = Concatenate Strings(w468, "</mod_slow>" ("string"), "\r\n", "</XML>" ("string")) -> (→"XML String":string)
          }
        }
      }
    }
    n256 = Merge Errors(w177, w176, w161) -> (w174:errorcluster)
    n257 = Unbundle By Name(w174) -> ("status"=w180:bool)
    n258 = Or(x=w180, y="stop") -> (x .or. y?=w178:bool)
    n259 = node-c288() -> ()  [unwired: 1 in, 1 out]
  }
  n260 = node-c288(w20) -> ()  [unwired: 7 out]
  n261 = local read "Write to file"() -> (w9:bool)
  n262 = VISA Close(VISA resource name=w16, error in (no error)=w15) -> (error out=w17:errorcluster)
  n263 = case shown="True" w9 {
    tunnel: w12 -> [_ w528]
    tunnel: w11 -> [_ w527]
    tunnel: w3 -> [_ w526]
    tunnel: w1 -> [_ w522]
    frame False {
    }
    frame True {
      n264 = Close File(refnum=w528) -> ()  [unwired: 1 in, 2 out]
      n265 = Close File(refnum=w527) -> ()  [unwired: 1 in, 2 out]
      n266 = Close File(refnum=w526) -> ()  [unwired: 1 in, 2 out]
      n267 = local read "XML String"() -> (w524:string)
      n268 = call "UTF8 LV80.vi"("text"=w524) -> ("utf-8 text out"=w523:string)
      n269 = Write to Text File(file (use dialog)=w522, text=w523) -> (refnum out=w525:refnum<file>)  [unwired: 2 in, 2 out]
      n270 = Close File(refnum=w525) -> ()  [unwired: 1 in, 2 out]
    }
  }
  n271 = call <vilib>:"Simple Error Handler.vi"("error in (no error)"=w17) -> ()  [unwired: 1 in, 8 out]
